vi "lenght vlue.vi"() -> ()   [LabVIEW 2020]
uses:
  <vilib>/Instr/_visa.llb/VISA Configure Serial Port (Instr).vi
panel:
  out "output 2":dbl
  out "output 1":dbl
  out "String":string
  in  "VISA resource name":refnum<visa-resource-name>
  in  "stop":bool
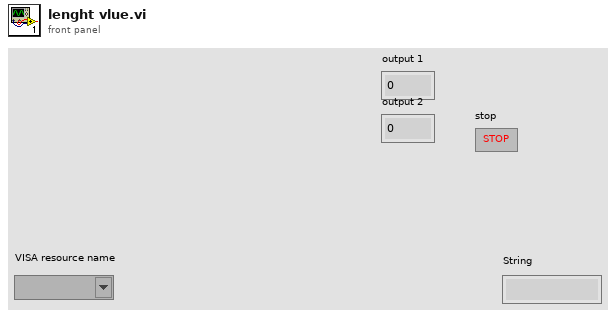
[diagram p1: front panel]
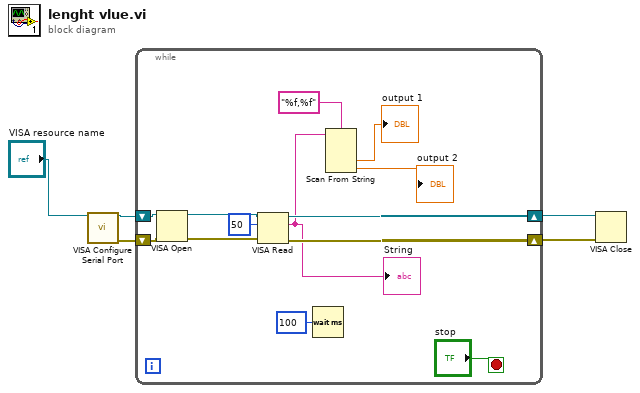
[diagram p0: block diagram]
diagram:
  n1 = call-poly "VISA Configure Serial Port"("VISA resource name"="VISA resource name") -> ("VISA resource name out"=w5:refnum<visa-resource-name>, "error out"=w3:errorcluster)  [unwired: 13 in]
  n2 = while {
    shift-right: [w16] -> w4
    shift-left: w5 -> [w18]
    shift-right: [w13] -> w2
    shift-left: w3 -> [w15]
    stop <- "stop" stop-if-true
    n3 = VISA Open(error in (no error)=w15, VISA resource name=w18) -> (VISA resource name=w17:refnum<visa-resource-name>, error out=w14:errorcluster)  [unwired: 3 in]
    n4 = VISA Read(VISA resource name=w17, byte count=u32 50, error in (no error)=w14) -> (VISA resource name out=w16:refnum<visa-resource-name>, read buffer=w9:string, error out=w13:errorcluster)  [unwired: 1 out]
    "String" <- w9
    n5 = Wait (ms)(milliseconds to wait=u32 100) -> ()  [unwired: 1 out]
    n6 = Scan From String(format string="%f,%f", input string=w9) -> (output 1=→"output 1":dbl, output 2=→"output 2":dbl)  [unwired: 4 in, 3 out]
  }
  n7 = VISA Close(VISA resource name=w4, error in (no error)=w2) -> ()  [unwired: 1 out]
